vi "template_WiFi_SSID.vi"   [LabVIEW 2014]
doc: "is a desing template VI for WiFi with fixed SSID application."
uses:
  QwaveSys_ESP8266/QwaveSys_ESP8266.lvlib
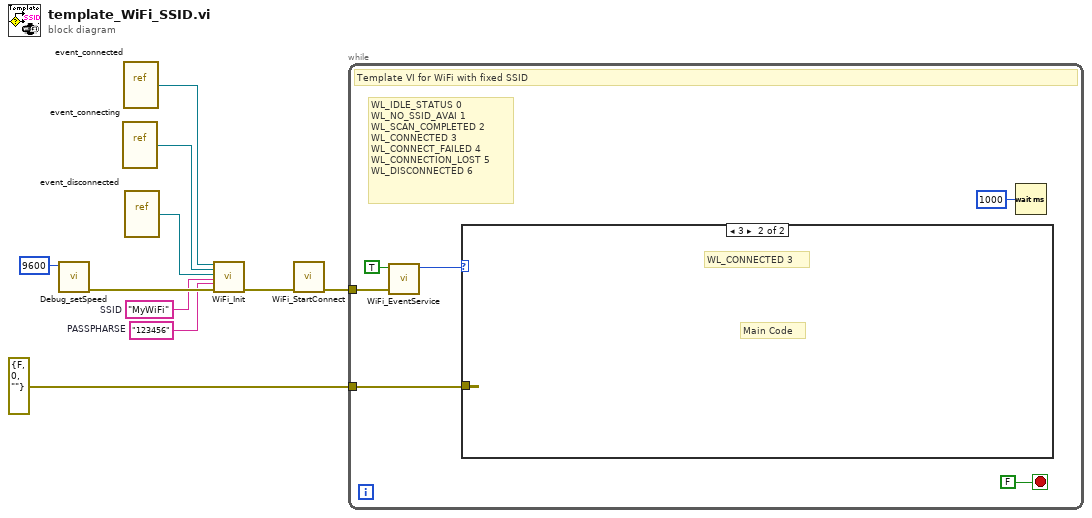
[diagram p0: block diagram]
diagram:
  w2 = "123456"  # PASSPHARSE
  w3 = "MyWiFi"  # SSID
  n1 = call "Debug_setSpeed.vi"("Speed"=u32 9600) -> ("error out"=w4:errorcluster)  [unwired: 10 in]
  n2 = vi-ref "event_connecting.vi"() -> (w9:refnum<vi>)
  n3 = vi-ref "event_connected.vi"() -> (w8:refnum<vi>)
  n4 = vi-ref "event_disconnected.vi"() -> (w7:refnum<vi>)
  n5 = call "WiFi_Init.vi"("connected"=w8, "connecting"=w9, "disconnected"=w7, "SSID"=w3, "PASSPHARSE"=w2, "error in (no error)"=w4) -> ("error out"=w5:errorcluster)  [unwired: 9 in]
  n6 = call "WiFi_StartConnect.vi"("error in (no error)"=w5) -> ("error out"=w10:errorcluster)  [unwired: 10 in]
  n7 = while {
    tunnel: w10 -> [w15]
    tunnel: errorcluster {"status"=FALSE, "code"=0, "source"=""} ("error out") -> [w11]
    stop <- FALSE stop-if-true
    # "WL_IDLE_STATUS\t0\nWL_NO_SSID_AVAI\t1\nWL_SCAN_COMPLETED\t2\nWL_CONNECTED\t3\nWL_CONNECT_FAILED\t4\nWL_CONNECTION_LOST\t5\nWL_DISCONNECTED\t6"
    # "Template VI for WiFi with fixed SSID"
    n8 = call "WiFi_EventService.vi"("error in (no error)"=w15, "wait for connected (True)"=TRUE) -> ("Status"=w12:u16)  [unwired: 8 in, 1 out]
    n9 = case shown="3" w12 {
      tunnel: w11 -> [_ _]
      frame 0, Default {
        # "DISCONNECTED or default status"
      }
      frame 3 {
        # "WL_CONNECTED\t3"
        # "Main Code"
      }
    }
    n10 = Wait (ms)(milliseconds to wait=u32 1000) -> ()  [unwired: 1 out]
  }
